vi "Size.vi"(8 "error in (no error)":errorcluster, 11 "Boolean Array in":refnum<class "Boolean Array.lvclass">) -> (0 "error out":errorcluster, 2 "Size":i32, 3 "Boolean Array out":refnum<class "Boolean Array.lvclass">)   [LabVIEW 2020, in "Data.lvlib" / "Boolean Array.lvclass"]
doc: "Return the size of the generic data element."
uses:
  Boolean Array.lvclass
  Boolean Array.lvclass/Boolean Array.ctl
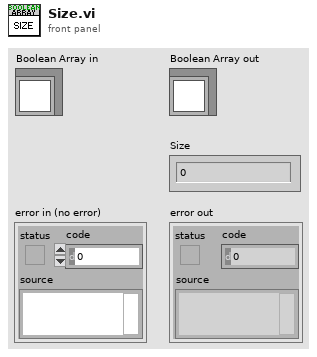
[diagram p1: front panel]
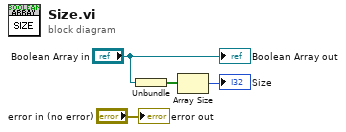
[diagram p0: block diagram]
diagram:
  n1 = Unbundle("Boolean Array in") -> (w2:bool[])
  n2 = Array Size(array=w2) -> (size(s)=→"Size":i32)
  "error out" <- "error in (no error)"
  "Boolean Array out" <- "Boolean Array in"
